vi "F206_Simple_Test1.vi"(0 "System no.":i32=1 min=1 max=4 step=1, 2 "How many additional axes?":u16(ring) items=["None", "One axis (A)", "Two axes (A and B)"], 4 "Is a NanoCube present?":bool, 5 "error in":errorcluster, 6 "Interface":u16(ring) items=["RS232", "GPIB"], 7 "Timeout":u32=5000, 8 "RS232 settings":cluster{"Portnumber":u16, "Baudrate":u16}={"Portnumber"=0, "Baudrate"=4} {"Baudrate" items=["9600", "14400", "19200", "38400", "57600", "115200"]; "Portnumber" items=["COM1", "COM2", "COM3", "COM4", "COM5", "COM6", "COM7", "COM8", "COM9"]}, 9 "GPIB settings":cluster{"Bus":i32, "Address":i32}={"Bus"=0, "Address"=4}) -> (14 "Identification":string, 16 "Conn. Axes":string[](array[string]), 19 "error out":errorcluster)   [LabVIEW 2011]
doc: "This simple test VI is a stand-alone sample application. \nSelect \nØ System number (= 1 in a one-system configuration),\nØ F-206 interface, \nØ timeout value, \nØ interface settings \nØ if any additional axes are connected to the F-206 controller, \nØ and if a NanoCube is connected to the F-206 controller,\nthen start the VI. The VI will open the chosen port and query for the identification (*IDN?) and help string (HELP). Depending on the chosen value of How many additional axes? and Is a NanoCube present? the connected axes ID's are returned. The diagram shows how to combine the driver VIs for these tasks."
uses:
  F206_V4.1.0/GCS_LabVIEW/Low Level/Communication.llb/Global1.vi
panel:
  # "Simple F-206 communication test program"
  # "Select F-206 interface, timeout value and interface settings, how many additional axes are connected to the F-206 controller and if\na NanoCube is connected to the F-206 controller first, then start the VI. The VI will open the chosen port, define the connected axes \nand query for Identification (*IDN?) and help string (HELP). See VI and control/ indicator information for details."
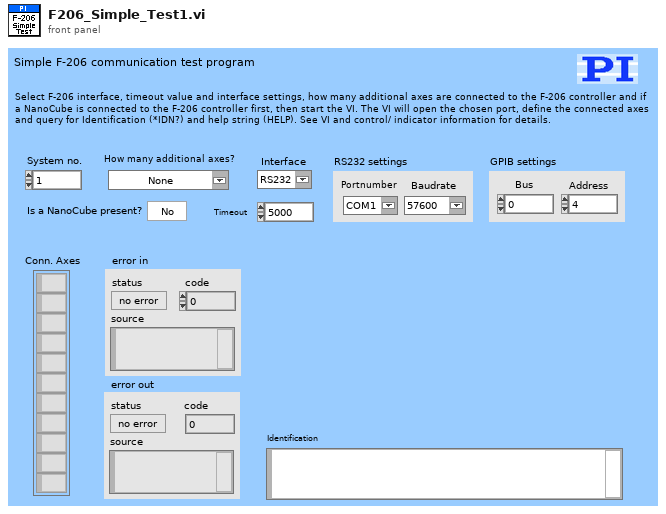
[diagram p1: front panel]
types:
  T1 = cluster{"RS232 Portnumber":u16, "Timeout":u32, "RS232 Baud rate":u32, "Interface":u16, "GPIB Bus":i32, "GPIB Address":i32, "GPIB Mode":i32}[]
  T2 = cluster{"input XON/XOFF":bool, "input HW Handshake":bool, "input alt HW HShk":bool, "output XON/XOFF":bool, "output HW Handshake":bool, "output alt HW HShk":bool, "XOFF byte ":u8, "XON byte":u8, "parity error byte":u16}[]
  T3 = cluster{"RS232 Portnumber":u16, "Timeout":u32, "RS232 Baud rate":u32, "Interface":u16, "GPIB Bus":i32, "GPIB Address":i32, "GPIB Mode":i32}
  T4 = cluster{"input XON/XOFF":bool, "input HW Handshake":bool, "input alt HW HShk":bool, "output XON/XOFF":bool, "output HW Handshake":bool, "output alt HW HShk":bool, "XOFF byte ":u8, "XON byte":u8, "parity error byte":u16}
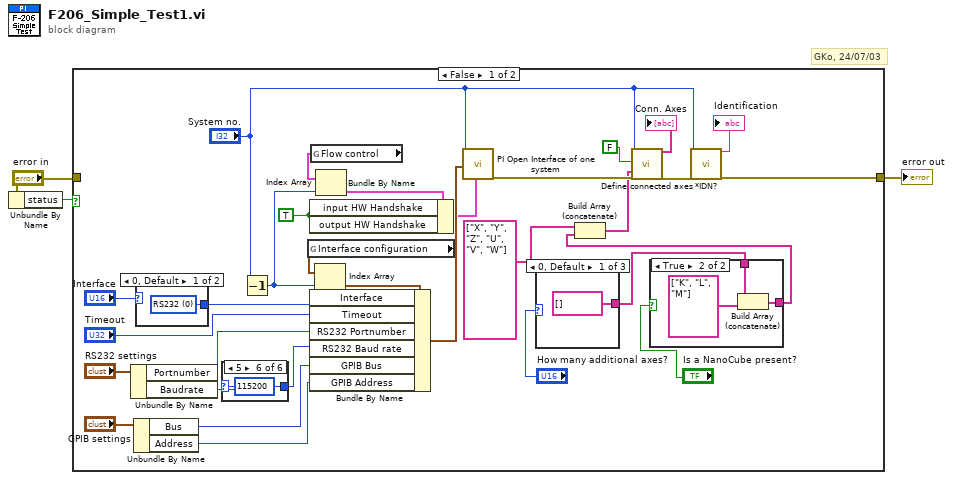
[diagram p0: block diagram]
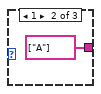
[diagram p3: hidden frame]
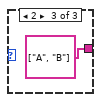
[diagram p4: hidden frame]
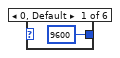
[diagram p5: hidden frame]
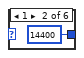
[diagram p6: hidden frame]
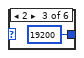
[diagram p7: hidden frame]
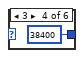
[diagram p8: hidden frame]
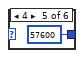
[diagram p9: hidden frame]
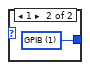
[diagram p10: hidden frame]
diagram:
  # "GKo, 24/07/03"
  n1 = Unbundle By Name("error in") -> ("status"=w1:bool)
  n2 = case shown="False" w1 {
    tunnel: [w4 w50] -> w2
    tunnel: "error in" -> [_ w50]
    frame False {
      w17 = TRUE ("Bundle Element")
      n3 = Unbundle By Name("RS232 settings") -> ("Portnumber"=w25:u16, "Baudrate"=w24:u16)
      n4 = Unbundle By Name("GPIB settings") -> ("Bus"=w21:i32, "Address"=w20:i32)
      n5 = case shown="0, Default" "Interface" {
        tunnel: [w48 w49] -> w28
        frame 0, Default {
          w48 = u16 0 items=["RS232", "GPIB", "DLL"] ("Interface")
        }
        frame 1 {
          w49 = u16 1 items=["RS232", "GPIB", "DLL"] ("Interface")
        }
      }
      n6 = case shown="5" w24 {
        tunnel: [9600 14400 19200 38400 57600 115200] -> w23
        frame 0, Default {
        }
        frame 1 {
        }
        frame 2 {
        }
        frame 3 {
        }
        frame 4 {
        }
        frame 5 {
        }
      }
      n7 = Decrement(x="System no.") -> (x-1=w15:i32)
      n8 = global read "Global1.vi" "Interface configuration"() -> (w19:T1)
      n9 = global read "Global1.vi" "Flow control"() -> (w16:T2)
      n10 = Index Array(array=w19, index=w15) -> (element=w30:T3)
      n11 = Bundle By Name(cluster=w30, "Interface"=w28, "Timeout"="Timeout", "RS232 Portnumber"=w25, "RS232 Baud rate"=w23, "GPIB Bus"=w21, "GPIB Address"=w20) -> (w14:T3)
      n12 = Index Array(array=w16, index=w15) -> (element=w18:T4)
      n13 = Bundle By Name(cluster=w18, "input HW Handshake"=w17, "output HW Handshake"=w17) -> (w13:T4)
      n14 = call "PI Open Interface of one system.vi"("System\nnumber"="System no.", "Interface configuration"=w14, "Flow control"=w13) -> ("error out"=w32:errorcluster)  [unwired: 16 in]
      n15 = case shown="0, Default" "How many additional axes?" {
        tunnel: [string[] [] string[] ["A"] string[] ["A", "B"]] -> w7
        frame 0, Default {
        }
        frame 1 {
        }
        frame 2 {
        }
      }
      n16 = case shown="True" "Is a NanoCube present?" {
        tunnel: [w35 w38] -> w5
        tunnel: w7 -> [w35 w36]
        frame False {
        }
        frame True {
          n17 = Build Array (concatenate)(w36, string[] ["K", "L", "M"]) -> (w38:string[])
        }
      }
      n18 = Build Array (concatenate)(string[] ["X", "Y", "Z", "U", "V", "W"] ("Conn. axes"), w5) -> (w8:string[])
      n19 = call "Define connected axes.vi"("System no."="System no.", "Read from\ncontroller?"=FALSE ("Read from\nController"), "Conn. axes"=w8, "error in"=w32) -> ("Conn. Axes out"=→"Conn. Axes":string[], "error out"=w12:errorcluster)  [unwired: 14 in]
      n20 = call "*IDN?.vi"("System no."="System no.", "error in"=w12) -> ("Identification"=→"Identification":string, "error out"=w4:errorcluster)  [unwired: 16 in]
    }
    frame True {
    }
  }
  "error out" <- w2
